vi "CoPilot Analyze.vi"(0 "JoystickDevRef":T1, 11 "Climbing Manual Enabled":bool) -> (2 "Go Manual":bool, 3 "Flipper Min":bool, 4 "auto shooting management":bool, 6 "Elevation":dbl, 8 "Shoot Motors":dbl, 10 "Flipper Max":bool, 13 "conveyer belt down":bool, 14 "conveyer belt up":bool, 15 "La Fire at will?":bool)   [LabVIEW 2012]
uses:
  <vilib>/Rock Robotics/WPI/Joystick/WPI_JoystickDevRef.ctl
  <vilib>/Rock Robotics/WPI/Joystick/WPI_JoystickDeviceEnum.ctl
  BotStatus.vi
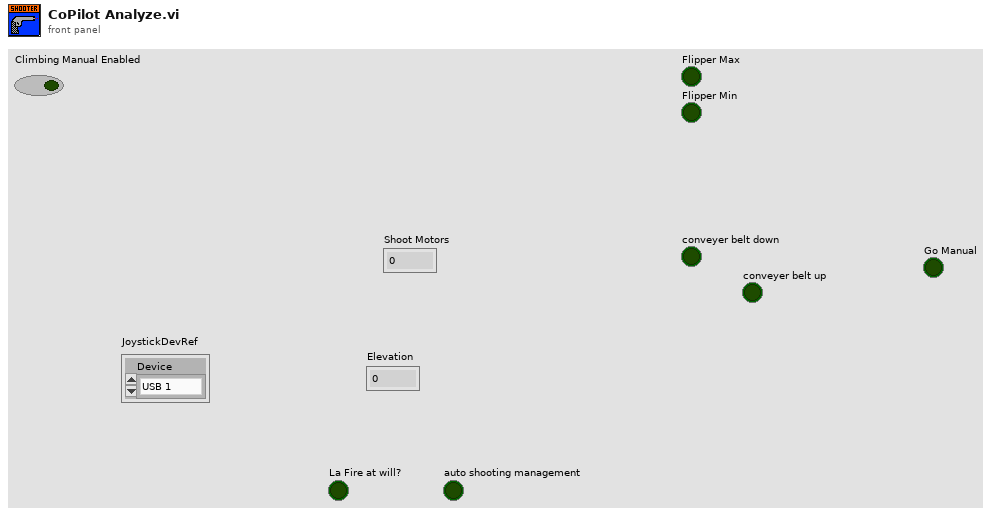
[diagram p1: front panel]
types:
  T1 = typedef "WPI_JoystickDevRef.ctl" = cluster{"Device":T2}
  T2 = typedef "WPI_JoystickDeviceEnum.ctl" = enum16{"USB 1", "USB 2", "USB 3", "USB 4", "Kinect 1", "Kinect 2"}
  T3 = typedef "WPI_JoystickButtonState.ctl" = cluster{"Button 1":bool, "Button 2":bool, "Button 3":bool, "Button 4":bool, "Button 5":bool, "Button 6":bool, "Button 7":bool, "Button 8":bool, "Button 9":bool, "Button 10":bool, "Button 11":bool, "Button 12":bool}
  T4 = cluster{"axis 1 (x)":dbl, "axis 2 (y)":dbl, "axis 3 (throttle)":dbl, "axis 4":dbl, "axis 5":dbl, "axis 6":dbl}
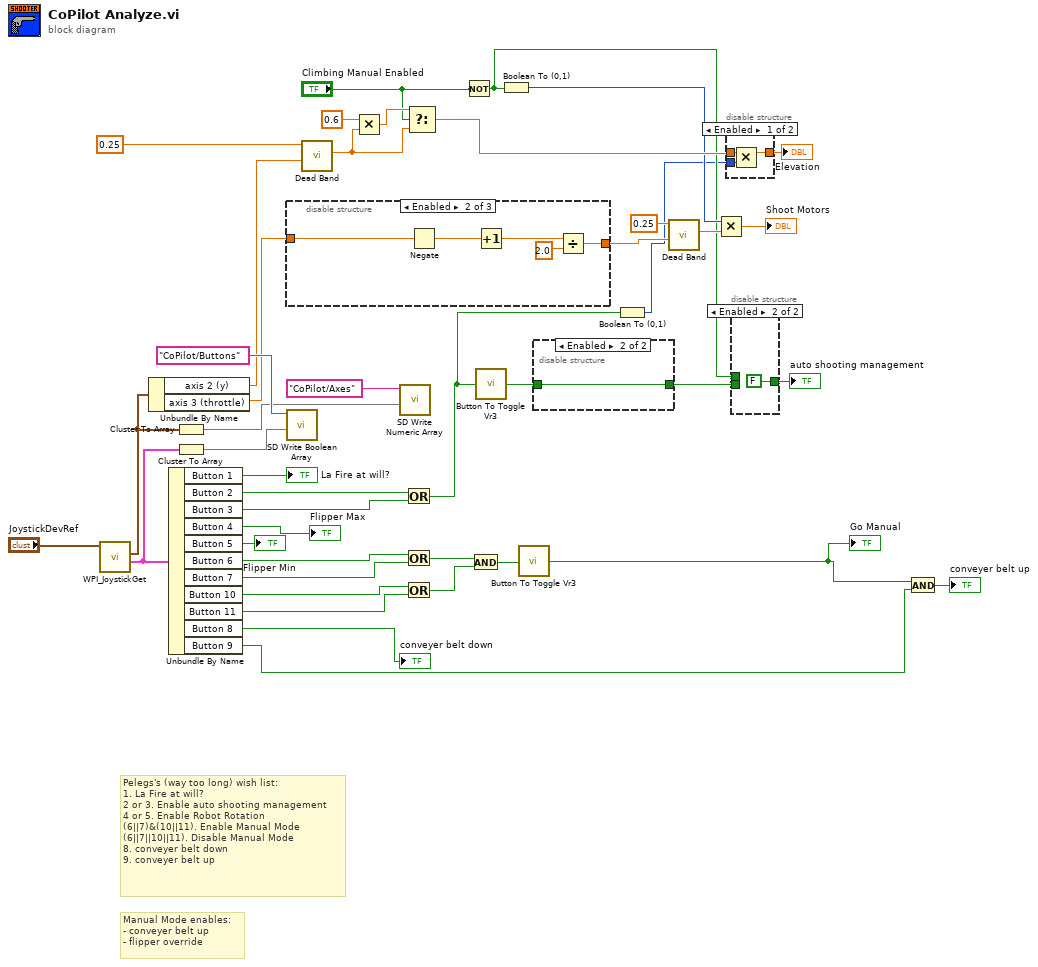
[diagram p0: block diagram]
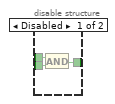
[diagram p3: hidden frame]
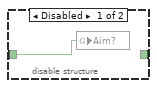
[diagram p4: hidden frame]
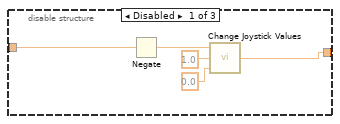
[diagram p5: hidden frame]
diagram:
  # "Manual Mode enables:\n- conveyer belt up\n- flipper override"
  # "Pelegs's (way too long) wish list:\n1. La Fire at will?\n2 or 3. Enable auto shooting management\n4 or 5. Enable Robot Rotation\n(6||7)&(10||11). Enable Manual Mode\n(6||7||10||11). Disable Manual Mode\n8. conveyer belt down\n9. conveyer belt up"
  n1 = call <vilib>:"WPI_JoystickGet.vi"("JoystickDevRef"="JoystickDevRef") -> ("Buttons"=w17:T3, "Axes"=w38:T4)  [unwired: 4 in, 1 out]
  n2 = Unbundle By Name(w38) -> ("axis 2 (y)"=w36:dbl, "axis 3 (throttle)"=w33:dbl)
  n3 = Unbundle By Name(w17) -> ("Button 1"=→"La Fire at will?":bool, "Button 2"=w30:bool, "Button 3"=w29:bool, "Button 4"=→"Flipper Max":bool, "Button 5"=→"Flipper Min":bool, "Button 6"=w28:bool, "Button 7"=w27:bool, "Button 10"=w26:bool, "Button 11"=w25:bool, "Button 8"=→"conveyer belt down":bool, "Button 9"=w19:bool)
  n4 = Cluster To Array(cluster=w38) -> (array=w40:dbl[])
  n5 = Cluster To Array(cluster=w17) -> (array=w42:bool[])
  n6 = disable-structure shown="Enabled" {
    disable-tunnel: w33 -> [w45 w53 w54]
    disable-tunnel: [w48 w50 w54] -> w32
    frame Disabled {
      n7 = Negate(x=w45) -> (-x=w44:dbl)
      n8 = call "Change Joystick Values.vi"("Change -1 to?"=0.0, "Change 1 to?"=1.0, "Joystick Input"=w44) -> ("Output Value"=w48:dbl)
    }
    frame Enabled {
      n9 = Negate(x=w53) -> (-x=w49:dbl)
      n10 = Increment(x=w49) -> (x+1=w52:dbl)
      n11 = Divide(x=w52, y=2.0) -> (x/y=w50:dbl)
    }
    frame Disabled {
    }
  }
  n12 = call <vilib>:"SD Write Boolean Array.vi"("Boolean Array"=w42, "Name"="CoPilot/Buttons") -> ()  [unwired: 8 in, 2 out]
  n13 = call "Dead Band.vi"("Axis In"=w36, "Dead Band"=0.25) -> ("Axis Out"=w14:dbl)  [unwired: 9 in]
  n14 = Multiply(x=0.6, y=w14) -> (x*y=w15:dbl)
  n15 = call <vilib>:"SD Write Numeric Array.vi"("Numeric Array"=w40, "Name"="CoPilot/Axes") -> ()  [unwired: 8 in, 2 out]
  n16 = Or(x=w30, y=w29) -> (x .or. y?=w4:bool)
  n17 = Or(x=w28, y=w27) -> (x .or. y?=w24:bool)
  n18 = Or(x=w26, y=w25) -> (x .or. y?=w23:bool)
  n19 = Select(t=w15, s="Climbing Manual Enabled", f=w14) -> (s? t:f=w13:dbl)
  n20 = Not(x="Climbing Manual Enabled") -> (.not. x?=w8:bool)
  n21 = And(x=w24, y=w23) -> (x .and. y?=w2:bool)
  n22 = call "Button To Toggle Vr3.vi"("InValue"=w4) -> ("Result"=w20:bool)
  n23 = Boolean To (0,1)(Boolean=w8) -> (0, 1=w10:i16)
  n24 = call "Button To Toggle Vr3.vi"("InValue"=w2) -> ("Result"=w1:bool)
  "Go Manual" <- w1
  n25 = disable-structure shown="Enabled" {
    disable-tunnel: w20 -> [w55 w56]
    disable-tunnel: [_ w56] -> w31
    frame Disabled {
      n26 = global write "BotStatus.vi" "Aim?"(w55) -> ()
    }
    frame Enabled {
    }
  }
  n27 = Boolean To (0,1)(Boolean=w4) -> (0, 1=w3:i16)
  n28 = call "Dead Band.vi"("Axis In"=w32, "Dead Band"=0.25) -> ("Axis Out"=w21:dbl)  [unwired: 9 in]
  n29 = Multiply(x=w10, y=w21) -> (x*y=→"Shoot Motors":dbl)
  n30 = disable-structure shown="Enabled" {
    disable-tunnel: w13 -> [w59 w60]
    disable-tunnel: [w58 w60] -> w5
    disable-tunnel: w3 -> [w57 _]
    frame Enabled {
      n31 = Multiply(x=w59, y=w57) -> (x*y=w58:dbl)
    }
    frame Disabled {
    }
  }
  "Elevation" <- w5
  n32 = disable-structure shown="Enabled" {
    disable-tunnel: w31 -> [w63 _]
    disable-tunnel: [w62 FALSE ("auto shooting management")] -> w9
    disable-tunnel: w8 -> [w61 _]
    frame Disabled {
      n33 = And(x=w61, y=w63) -> (x .and. y?=w62:bool)
    }
    frame Enabled {
    }
  }
  "auto shooting management" <- w9
  n34 = And(x=w1, y=w19) -> (x .and. y?=→"conveyer belt up":bool)
